vi "DSF.Engine.Interface.Builder.Destroy.vi"(8 "error in (no error)":errorcluster, 11 "Builder Interface in":refnum<class "DSF.Engine.Interface.Builder.lvclass">) -> (0 "error out":errorcluster)   [LabVIEW 2016, in "DSF.Engine.lvlib" / "DSF.Engine.Interface.Builder.lvclass"]
uses:
  DSF.Engine.Interface.Builder.lvclass
  C:/Git/Sourcetree/DSF/Source/Engine/Classes/Interface/DSF.Engine.Interface.lvclass
  DSF.Engine.Interface.lvclass/DSF.Engine.Interface.ctl
  DSF.Engine.Interface.Get Response FIFO.vi
  DSF.Engine.Interface.Get Command FIFO.vi
  DSF.Engine.Interface.RT FIFO.Delete.vi
  DSF.Engine.Interface.lvclass
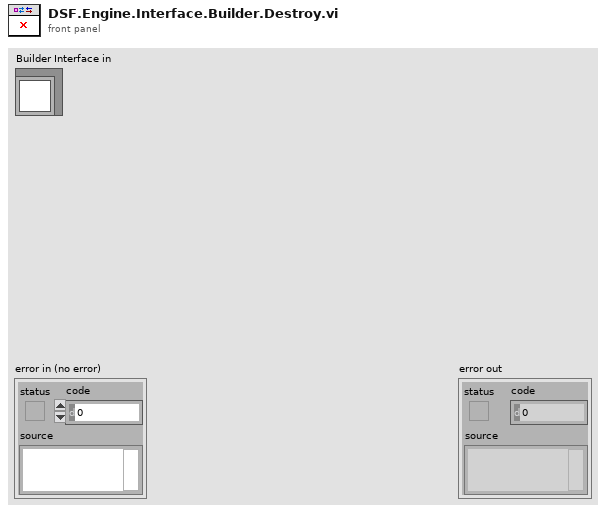
[diagram p1: front panel]
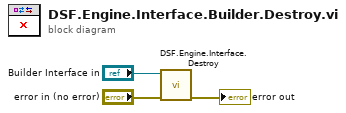
[diagram p0: block diagram]
diagram:
  n1 = call "DSF.Engine.Interface.Destroy.vi"("error in (no error)"="error in (no error)", "Interface in"="Builder Interface in") -> ("error out"=→"error out":errorcluster)  [unwired: 8 in, 1 out]
